vi "SSM.vi"(8 "Stopp":bool, 10 "SLOT":i32=100 min=0 max=999 step=100 format="%03d", 11 "USB":i32) -> ()   [LabVIEW 2020]
doc: "This VI provides a GUI for SSM modules. It implements an abstract module interface, where callers provide the only necessary and sufficient information for callee modules via the datafields USB, SLOT and Stopp. All module intern information are handled hidden by the module. Thereby, a caller must not \"know\" about such internals."
panel:
  in  "TriggerLevel [mV]":i32=421 min=-5000 max=5000 step=50 format="%5d"
  out "NeedsTrigLvl":bool[](array[boolean])
  in  "Trigger Source":i32(ring) items=["off", "40 MHz (int.)", "20 MHz (int.)", "10 MHz (int.)", "5 MHz (int.)", "2.5 MHz (int.)", "NIM (ext.)", "rising (ext.)", "falling (ext.)"]
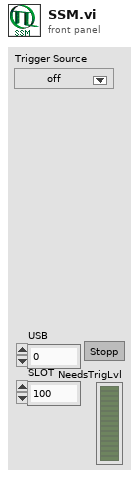
[diagram p1: front panel]
types:
  T1 = cluster{"MainFreqTrig":string, "MainFreq":i32, "TrigLevelEnabled":u8}[]
  T2 = cluster{"UpperTL":i32, "LowerTL":i32, "ResolTL":i32}
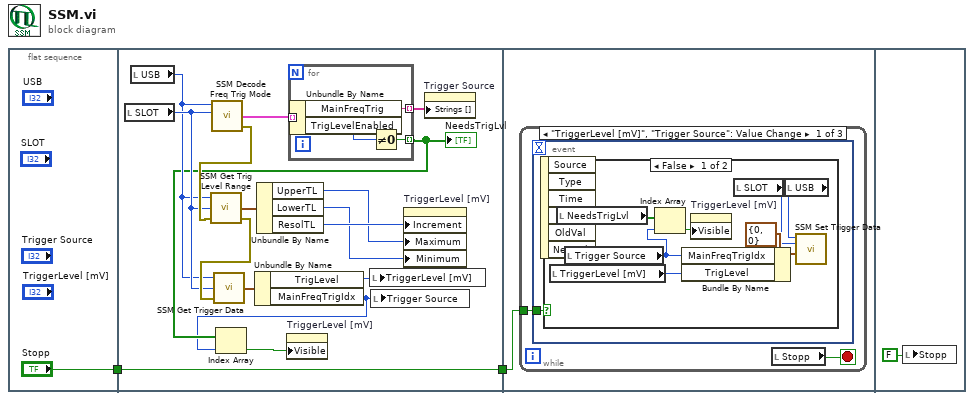
[diagram p0: block diagram]
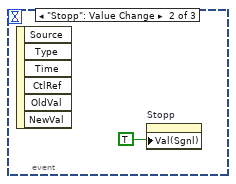
[diagram p3: hidden frame]
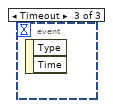
[diagram p4: hidden frame]
diagram:
  n1 = flat-sequence {
    tunnel: ["Stopp"] -> w1
    tunnel: [w4] -> w2
    tunnel: w1 -> [w4]
    tunnel: w2 -> [w24]
    frame #0 {
    }
    frame #1 {
      n2 = local read "SLOT"() -> (w13:i32)
      n3 = local read "USB"() -> (w12:i32)
      n4 = call "SSM Decode Freq Trig Mode.vi"("DevIdx"=w12, "SlotId"=w13) -> ("SSM Trigger Mode"=w18:T1, "error out"=w16:errorcluster)  [unwired: 3 in, 1 out]
      n5 = call "SSM Get Trig Level Range.vi"("error in (no error)"=w16, "SlotId"=w13, "DevIdx"=w12) -> ("error out"=w15:errorcluster, "SSM Trig Level Range"=w14:T2)  [unwired: 1 out]
      n6 = call "SSM Get Trigger Data.vi"("error in (no error)"=w15, "SlotId"=w13, "DevIdx"=w12) -> ("SSM Trigger Data"=w19:cluster{"MainFreqTrigIdx":i32, "TrigLevel":i32})  [unwired: 2 out]
      n7 = Unbundle By Name(w19) -> ("TrigLevel"=w7:i32, "MainFreqTrigIdx"=w6:i32)
      n8 = Unbundle By Name(w14) -> ("UpperTL"=w9:i32, "LowerTL"=w10:i32, "ResolTL"=w11:i32)
      n9 = for {
        tunnel: w18 -> [w23] mode=indexing
        tunnel: [w22] -> w17 mode=indexing
        tunnel: [w21] -> w8 mode=indexing
        n10 = Unbundle By Name(w23) -> ("MainFreqTrig"=w22:string, "TrigLevelEnabled"=w20:u8)
        n11 = Not Equal To 0?(x=w20) -> (x != 0?=w21:bool)
      }
      "NeedsTrigLvl" <- w8
      n12 = Index Array(array=w8, index=w6) -> (element=w5:bool)
      n13 = property on="TriggerLevel [mV]" class="DigNum (strict)"("Visible"=w5) -> ()  [unwired: 2 in, 2 out]
      n14 = local write "TriggerLevel [mV]"(w7) -> ()
      n15 = local write "Trigger Source"(w6) -> ()
      n16 = property on="TriggerLevel [mV]" class="DigNum (strict)"("Increment"=w11, "Maximum"=w9, "Minimum"=w10) -> ()  [unwired: 2 in, 2 out]
      n17 = property on="Trigger Source" class="Ring (strict)"("Strings []"=w17) -> ()  [unwired: 2 in, 2 out]
    }
    frame #2 {
      n18 = while {
        tunnel: w24 -> [w25]
        stop <- w26 stop-if-true
        n19 = event shown="[0] \"TriggerLevel [mV]\", \"Trigger Source\": Value Change" {
          selector: _ -> [_ _ _]
          dyn-events: _ -> [_ _ _]
          timeout: _ -> [_ _ _]
          tunnel: w25 -> [w27 _ _]
          event "TriggerLevel [mV]", "Trigger Source": Value Change {
            n20 = event-data() -> ()  [unwired: 1 in, 6 out]
            n21 = case shown="False" w27 {
              frame False {
                n22 = local read "TriggerLevel [mV]"() -> (w34:i32)
                n23 = local read "NeedsTrigLvl"() -> (w33:bool[])
                n24 = local read "Trigger Source"() -> (w35:i32)
                n25 = Index Array(array=w33, index=w35) -> (element=w32:bool)
                n26 = Bundle By Name(cluster=cluster{"MainFreqTrigIdx":i32, "TrigLevel":i32} {"MainFreqTrigIdx"=0, "TrigLevel"=0} ("SSM Trigger Data"), "MainFreqTrigIdx"=w35, "TrigLevel"=w34) -> (w31:cluster{"MainFreqTrigIdx":i32, "TrigLevel":i32})
                n27 = property on="TriggerLevel [mV]" class="DigNum (strict)"("Visible"=w32) -> ()  [unwired: 2 in, 2 out]
                n28 = local read "SLOT"() -> (w28:i32)
                n29 = local read "USB"() -> (w29:i32)
                n30 = call "SSM Set Trigger Data.vi"("SSM Trigger Data"=w31, "SlotId"=w28, "DevIdx"=w29) -> ()  [unwired: 1 in, 2 out]
              }
              frame True {
              }
            }
          }
          event "Stopp": Value Change {
            n31 = event-data() -> ()  [unwired: 1 in, 6 out]
            n32 = property on="Stopp" class="Bool (strict)"("Val(Sgnl)"=TRUE ("Value (Signaling)")) -> ()  [unwired: 2 in, 2 out]
          }
          event Timeout {
            n33 = event-data() -> ()  [unwired: 1 in, 2 out]
          }
        }
        n34 = local read "Stopp"() -> (w26:bool)
      }
    }
    frame #3 {
      n35 = local write "Stopp"(FALSE ("Stopp")) -> ()
    }
  }
